vi "DuelistRole.vi"(7 "firstCall":bool=TRUE, 8 "error in (no error)":errorcluster, 9 "RobotRef":refnum<class "Robot.lvclass">, 10 "Game in":refnum<class "Game.lvclass">, 11 "DuelistRole in":refnum<class "DuelistRole.lvclass">) -> (0 "error out":errorcluster, 2 "Robot out":refnum<class "Robot.lvclass">, 3 "DuelistRole out":refnum<class "DuelistRole.lvclass">)   [LabVIEW 2020, in "DuelistRole.lvclass"]
uses:
  DuelistRole.lvclass
  C:/Users/Administrator/Desktop/SSL/SSL_AI/Role_class/Role.lvclass
  Robot_class/Robot.lvclass
  Game_class/Game.lvclass
  Role_class/Role.lvclass/Role.ctl
  ShootTactic_class/States.ctl
  Tacticbook_class/Tacticbook.lvclass/Tacticbook.ctl
  ShootTactic_class/ShootTactic.lvclass/ShootTactic.ctl
  Tacticbook_class/Read ShootTactic.vi
  ShootTactic_class/Read States.vi
  Tacticbook_class/Write ShootTactic.vi
  Role_class/Read Tacticbook.vi
  Role_class/Read tactic_index.vi
  Role_class/Write Tacticbook.vi
  Role_class/Write tactic_index.vi
  Tacticbook_class/Tacticbook.lvclass
  ShootTactic_class/ShootTactic.lvclass
panel:
  out "Game out":refnum<class "Game.lvclass">
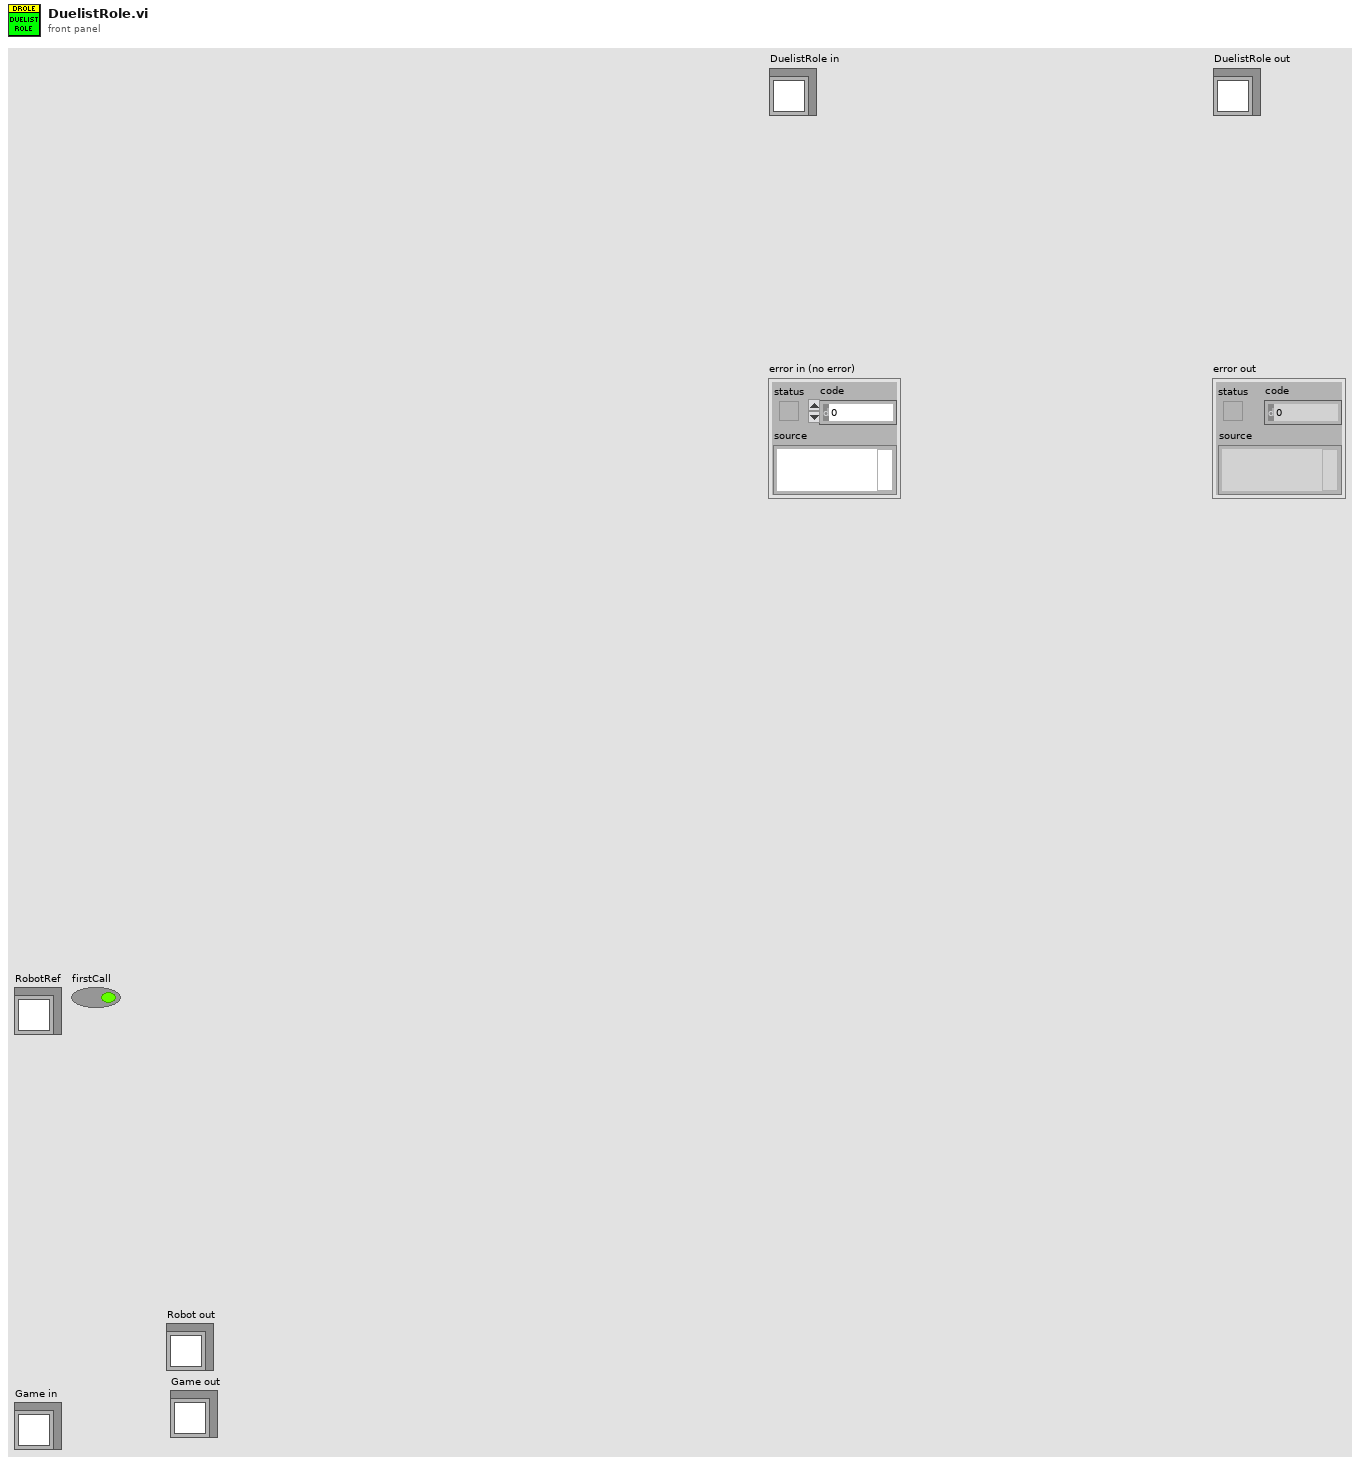
[diagram p1: front panel]
types:
  T1 = typedef "ShootTactic.lvclass/States.ctl" = enum16{"BallInGoalieArea", "Exit", "KickToGoal", "StealBall"}
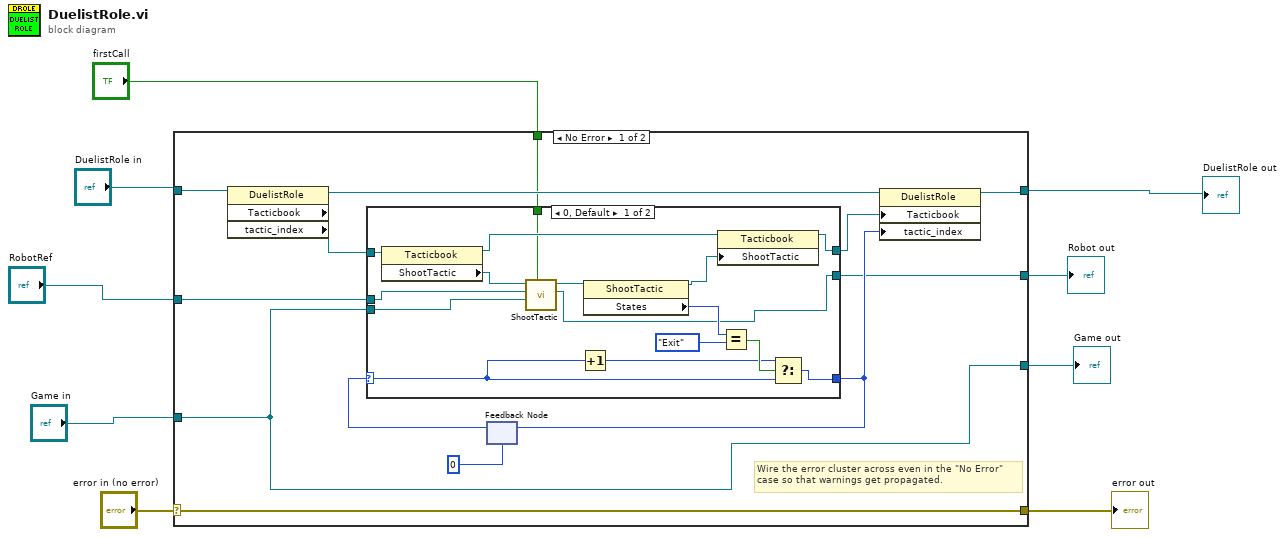
[diagram p0: block diagram]
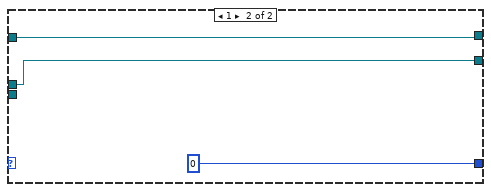
[diagram p2: hidden frame]
diagram:
  n1 = case shown="No Error" "error in (no error)" {
    selector: "error in (no error)" -> [w22 w45]
    tunnel: [w22 w45] -> w3
    tunnel: [w20 w44] -> w5
    tunnel: "DuelistRole in" -> [w21 w44]
    tunnel: "RobotRef" -> [w14 w43]
    tunnel: [w13 w43] -> w9
    tunnel: [w11 w42] -> w8
    tunnel: "Game in" -> [w11 w42]
    tunnel: "firstCall" -> [w10 _]
    frame No Error {
      # "Wire the error cluster across even in the \"No Error\"\ncase so that warnings get propagated."
      n2 = property class="DuelistRole" props=["Tacticbook", "tactic_index"](reference=w21) -> (reference out=w19:refnum<class "DuelistRole.lvclass">, "Tacticbook"=w16:refnum<class "Tacticbook.lvclass">)  [unwired: 1 in, 2 out]
      n3 = feedback #1(0) -> (w17:i32)
      n4 = case shown="0, Default" w17 {
        selector: w17 -> [w35 _]
        tunnel: [w36 0] -> w15
        tunnel: w16 -> [w38 w39]
        tunnel: w14 -> [w26 w41]
        tunnel: [w27 w41] -> w13
        tunnel: [w32 w39] -> w12
        tunnel: w11 -> [w25 _]
        tunnel: w10 -> [w23 _]
        frame 0, Default {
          n5 = property class="Tacticbook"(reference=w38) -> (reference out=w33:refnum<class "Tacticbook.lvclass">, "ShootTactic"=w31:refnum<class "ShootTactic.lvclass">)  [unwired: 1 in, 1 out]
          n6 = call "ShootTactic.vi"("firstCall"=w23, "Game in"=w25, "Robot"=w26, "ShootTactic in"=w31) -> ("Robot out"=w27:refnum<class "Robot.lvclass">, "ShootTactic out"=w30:refnum<class "ShootTactic.lvclass">)  [unwired: 5 in, 1 out]
          n7 = Increment(x=w35) -> (x+1=w34:i32)
          n8 = property class="ShootTactic"(reference=w30) -> (reference out=w29:refnum<class "ShootTactic.lvclass">, "States"=w28:T1)  [unwired: 1 in, 1 out]
          n9 = property class="Tacticbook"(reference=w33, "ShootTactic"=w29) -> (reference out=w32:refnum<class "Tacticbook.lvclass">)  [unwired: 1 in, 1 out]
          n10 = Equal?(x=w28, y=States."Exit") -> (x = y?=w37:bool)
          n11 = Select(t=w34, s=w37, f=w35) -> (s? t:f=w36:i32)
        }
        frame 1 {
        }
      }
      n12 = feedback-in #1(w15) -> ()
      n13 = property class="DuelistRole"(reference=w19, "Tacticbook"=w12, "tactic_index"=w15) -> (reference out=w20:refnum<class "DuelistRole.lvclass">)  [unwired: 1 in, 1 out]
    }
    frame Error {
    }
  }
  "error out" <- w3
  "DuelistRole out" <- w5
  "Robot out" <- w9
  "Game out" <- w8
